vi "VI_WithGlobalDAQmxTask.vi"(11 "DAQmx Task Name":refnum<k21>="MyVoltageTask") -> (3 "DAQmx Task Out":refnum<k21>)   [LabVIEW 2012]
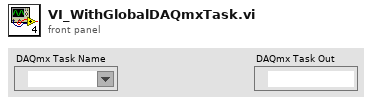
[diagram p1: front panel]
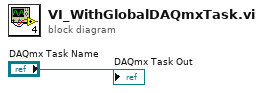
[diagram p0: block diagram]
diagram:
  "DAQmx Task Out" <- "DAQmx Task Name"
